vi "S-Curve Goal to Velocity.vi"(6 "g":dbl, 8 "c2":dbl, 9 "c1":dbl, 10 "a":dbl, 11 "x":dbl) -> (3 "v":dbl)   [LabVIEW 2020]
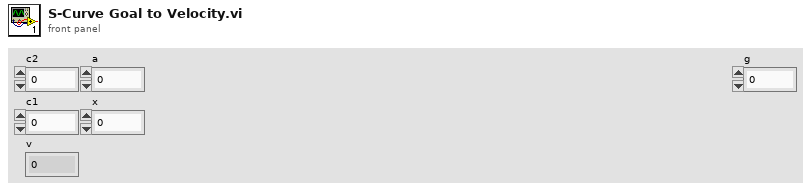
[diagram p1: front panel]
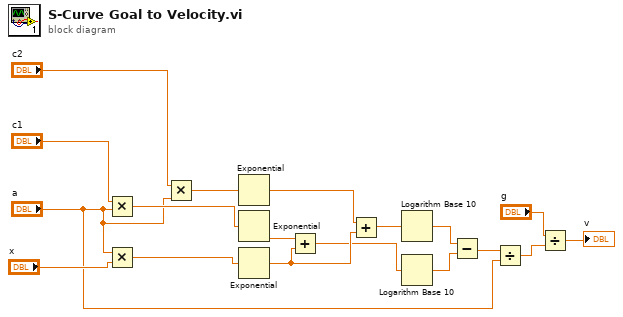
[diagram p0: block diagram]
diagram:
  n1 = Multiply(x="c1", y="a") -> (x*y=w14:dbl)
  n2 = Multiply(x="a", y="x") -> (x*y=w13:dbl)
  n3 = Multiply(x="c2", y="a") -> (x*y=w15:dbl)
  n4 = Exponential(1:w15) -> (0:w11:dbl)
  n5 = Exponential(1:w14) -> (0:w12:dbl)
  n6 = Exponential(1:w13) -> (0:w10:dbl)
  n7 = Add(x=w12, y=w10) -> (x+y=w8:dbl)
  n8 = Add(x=w11, y=w10) -> (x+y=w9:dbl)
  n9 = Logarithm Base 10(1:w9) -> (0:w7:dbl)
  n10 = Logarithm Base 10(1:w8) -> (0:w6:dbl)
  n11 = Subtract(x=w7, y=w6) -> (x-y=w5:dbl)
  n12 = Divide(x=w5, y="a") -> (x/y=w3:dbl)
  n13 = Divide(x="g", y=w3) -> (x/y=→"v":dbl)
